vi "Mixer.Show.vi"() -> (0 "success":bool)   [LabVIEW 2020]
uses:
  <vilib>/Utility/sysdir.llb/System Directory Type.ctl
  <vilib>/Utility/config.llb/Read Key (I32).vi
  SubVIs/Mixer.Globals.vi
  <vilib>/Utility/config.llb/NI_LVConfig.lvlib
panel:
  out "error out":errorcluster
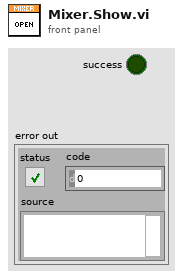
[diagram p1: front panel]
types:
  T1 = enum32{"Bad", "Idle", "Run top level", "Running"}
  T2 = enum32{"Invalid", "Standard", "Closed", "Hidden", "Minimized", "Maximized"}
  T3 = typedef "System Directory Type.ctl" = i32
  T4 = typedef "NI_LVConfig.lvlib/Config Data RefNum.ctl" = refnum<k1>
  T5 = typedef "LVRectTypeDef.ctl" = cluster{"Left":i16, "Top":i16, "Right":i16, "Bottom":i16}
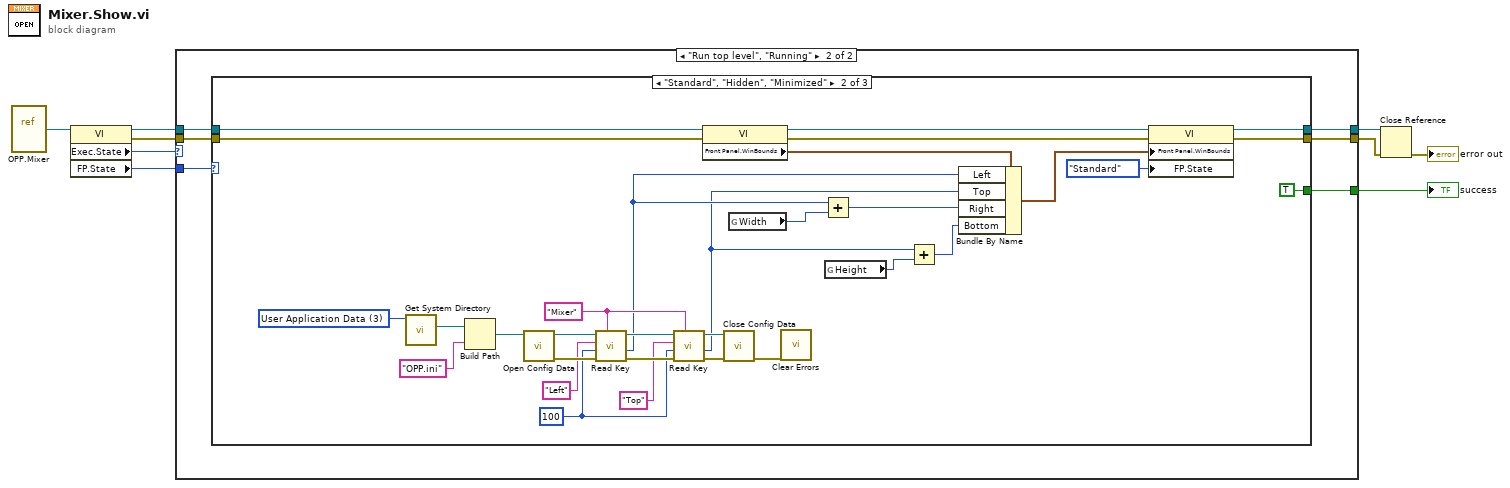
[diagram p0: block diagram]
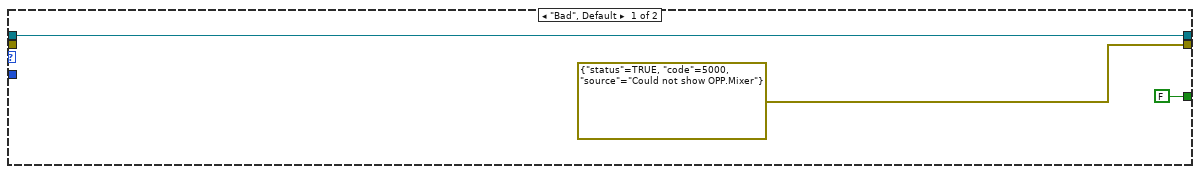
[diagram p2: hidden frame]
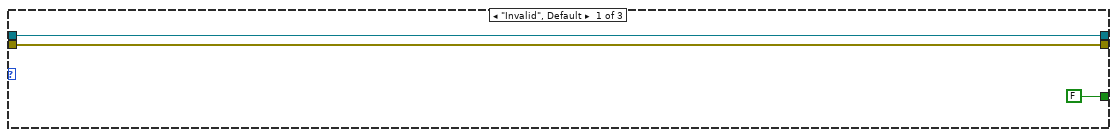
[diagram p3: hidden frame]
diagram:
  n1 = vi-ref "OPP.Mixer.vi"() -> (w5:refnum<vi>)
  n2 = property class="VI"(reference=w5) -> (reference out=w9:refnum<vi>, error out=w8:errorcluster, "Exec.State"=w3:T1, "FP.State"=w2:T2)  [unwired: 1 in]
  n3 = case shown="\"Run top level\", \"Running\"" w3 {
    tunnel: w9 -> [w12 w18]
    tunnel: w8 -> [_ w17]
    tunnel: [w12 w16] -> w7
    tunnel: [errorcluster {"status"=TRUE, "code"=5000, "source"="Could not show OPP.Mixer"} ("error out") w15] -> w6
    tunnel: w2 -> [_ w14]
    tunnel: [FALSE w13] -> w1
    frame "Bad", Default {
    }
    frame "Run top level", "Running" {
      n4 = case shown="\"Standard\", \"Hidden\", \"Minimized\"" w14 {
        tunnel: w18 -> [w21 w31 w54]
        tunnel: w17 -> [w20 w30 w53]
        tunnel: [w21 w27 w54] -> w16
        tunnel: [w20 w26 w53] -> w15
        tunnel: [FALSE TRUE _] -> w13
        frame "Invalid", Default {
        }
        frame "Standard", "Hidden", "Minimized" {
          w33 = 100 ("default value")
          w38 = "Mixer" ("section")
          w34 = T3 3 items=["User Home"=0, "User Desktop"=1, "User Documents"=2, "User Application Data"=3, "User Preferences"=4, "User Temporary"=5, "Public Documents"=6, "Public Application Data"=7, "Public Preferences"=8, "Public Cache"=13, "System Core Libraries"=9, "System Installed Libraries"=10, "Application Files"=11, "Boot Volume Root"=12] ("system directory type")
          n5 = call <vilib>:"Get System Directory.vi"("system directory type"=w34) -> ("system directory"=w46:path)  [unwired: 10 in]
          n6 = Build Path(base path=w46, name or relative path="OPP.ini") -> (appended path=w45:path)
          n7 = call <vilib>:"Open Config Data.vi"("configuration file path"=w45) -> ("error out"=w42:errorcluster, "refnum"=w44:T4)  [unwired: 8 in, 1 out]
          n8 = call-poly <vilib>:"Read Key.vi"("section"=w38, "error in (no error)"=w42, "default value"=w33, "key"="Left", "refnum"=w44) -> ("error out"=w41:errorcluster, "value"=w29:i32, "refnum out"=w43:T4)  [unwired: 3 in, 1 out]
          n9 = call-poly <vilib>:"Read Key.vi"("section"=w38, "error in (no error)"=w41, "default value"=w33, "key"="Top", "refnum"=w43) -> ("error out"=w40:errorcluster, "value"=w28:i32, "refnum out"=w39:T4)  [unwired: 3 in, 1 out]
          n10 = property class="VI"(reference=w31, error in=w30) -> (reference out=w49:refnum<vi>, error out=w48:errorcluster, "Front Panel.WinBounds"=w52:T5)
          n11 = call <vilib>:"Close Config Data.vi"("error in (no error)"=w40, "refnum"=w39) -> ("error out"=w32:errorcluster)  [unwired: 8 in, 1 out]
          n12 = global read "Mixer.Globals.vi" "Width"() -> (w23:i32)
          n13 = call <vilib>:"Clear Errors.vi"("error in (no error)"=w32) -> ()  [unwired: 5 in, 2 out]
          n14 = Add(x=w29, y=w23) -> (x+y=w51:i32)
          n15 = global read "Mixer.Globals.vi" "Height"() -> (w22:i32)
          n16 = Add(x=w28, y=w22) -> (x+y=w50:i32)
          n17 = Bundle By Name(cluster=w52, "Left"=w29, "Top"=w28, "Right"=w51, "Bottom"=w50) -> (w47:T5)
          n18 = property class="VI"(reference=w49, error in=w48, "Front Panel.WinBounds"=w47, "FP.State"=T2."Standard" ("Front Panel Window:State")) -> (reference out=w27:refnum<vi>, error out=w26:errorcluster)
        }
        frame "Closed" {
        }
      }
    }
  }
  "success" <- w1
  n19 = Close Reference(reference=w7, error in (no error)=w6) -> (error out=→"error out":errorcluster)
